vi "Read Data Increment.vi"(8 "error in (no error)":errorcluster, 11 "Data":refnum<class "Data.lvclass">) -> (0 "error out":errorcluster, 2 "dx":dbl format="%_6g", 3 "Data":refnum<class "Data.lvclass">)   [LabVIEW 2017, in "Data.lvclass"]
uses:
  <vilib>/addons/_NISVFA/_Shared subVIs/Data Objects/Data/Data.lvclass
  <vilib>/addons/_NISVFA/_Shared subVIs/Data Objects/Data/Data.lvclass/Data.ctl
  <vilib>/addons/_NISVFA/_Shared subVIs/Common/sv_Get NI Property Name String.vi
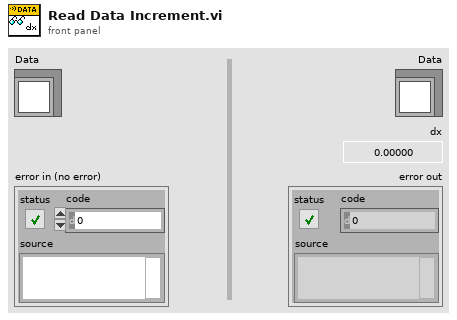
[diagram p1: front panel]
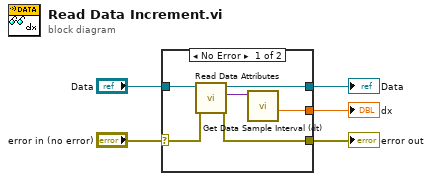
[diagram p0: block diagram]
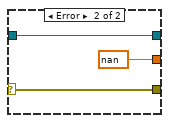
[diagram p2: hidden frame]
diagram:
  n1 = case shown="No Error" "error in (no error)" {
    selector: "error in (no error)" -> [w6 w12]
    tunnel: "Data" -> [w11 w14]
    tunnel: [w10 w14] -> w4
    tunnel: [w8 nan ("dt [s]")] -> w3
    tunnel: [w7 w12] -> w2
    frame No Error {
      n2 = call <vilib>:"Read Data Attributes.vi"("error in (no error)"=w6, "Data in"=w11) -> ("error out"=w7:errorcluster, "data attributes"=w9:variant, "Data out"=w10:refnum<class "Data.lvclass">)  [unwired: 7 in]
      n3 = call <vilib>:"Get Data Sample Interval (dt).vi"("variant in"=w9) -> ("dt [s]"=w8:dbl)  [unwired: 9 in, 1 out]
    }
    frame Error {
    }
  }
  "Data" <- w4
  "error out" <- w2
  "dx" <- w3
